vi "swap_inside_IPE.vi"(8 "error in (no error)":errorcluster, 10 "data bus in":T1, 11 "Test Data in":T2) -> (0 "error out":errorcluster, 2 "data bus out":T1, 3 "Test Data out":T2)   [LabVIEW 2024, in "IPE Optimization Tester.lvlib"]
uses:
  IPE Optimization Tester.lvlib
  test_data--cluster.ctl
  SubVIs/data_bus--cluster.ctl
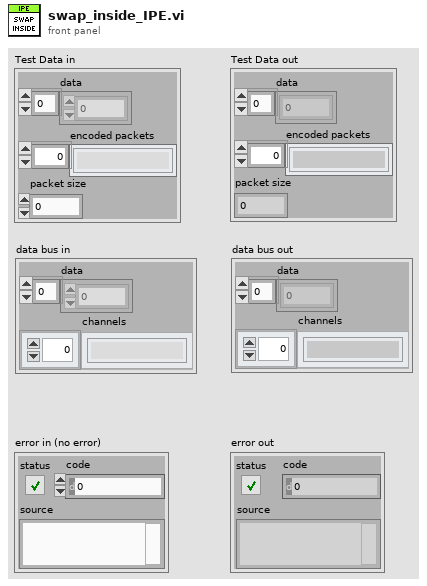
[diagram p1: front panel]
types:
  T1 = typedef "IPE Optimization Tester.lvlib/data_bus--cluster.ctl" = cluster{"data":dbl[], "channels":string[]}
  T2 = typedef "IPE Optimization Tester.lvlib/test_data--cluster.ctl" = cluster{"data":dbl[], "encoded packets":string[], "packet size":i32}
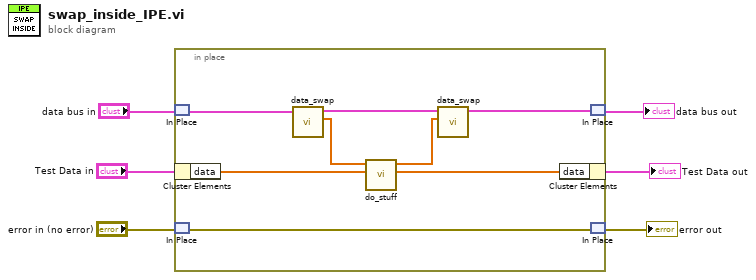
[diagram p0: block diagram]
diagram:
  n1 = in-place {
    n2 = in-place-match #1("data bus in") -> (w13:T1)
    n3 = in-place-cluster #2("Test Data in") -> ("data"=w10:dbl[])
    n4 = in-place-match #3("error in (no error)") -> (w14:errorcluster)
    n5 = call "data_swap.vi"("data bus in"=w13) -> ("data out"=w8:dbl[], "data bus out"=w12:T1)  [unwired: 9 in]
    n6 = call "do_stuff.vi"("live data in"=w10, "data bus in"=w8) -> ("live data out"=w9:dbl[], "data bus out"=w7:dbl[])  [unwired: 8 in]
    n7 = call "data_swap.vi"("data in"=w7, "data bus in"=w12) -> ("data bus out"=w11:T1)  [unwired: 8 in, 1 out]
    n8 = in-place-cluster #2("data"=w9) -> (→"Test Data out":T2)
    n9 = in-place-match #1(w11) -> (→"data bus out":T1)
    n10 = in-place-match #3(w14) -> (→"error out":errorcluster)
  }
